vi "tm_startrecorder.vi"(8 "error in (no error)":errorcluster, 9 "frames":i32, 10 "File":path, 11 "Handle in":u32) -> (0 "error out":errorcluster, 3 "Handle out":u32)   [LabVIEW 2023]
uses:
  tmcamcon.dll
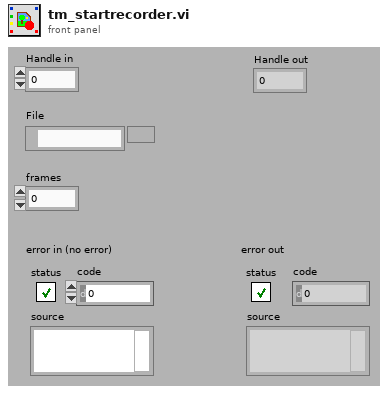
[diagram p1: front panel]
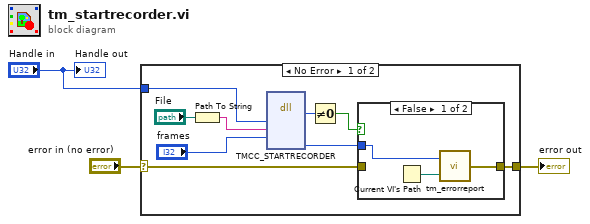
[diagram p0: block diagram]
diagram:
  n1 = case shown="No Error" "error in (no error)" {
    selector: "error in (no error)" -> [w7 w17]
    tunnel: [w4 w17] -> w2
    tunnel: "Handle in" -> [w11 _]
    frame No Error {
      n2 = Path To String(path="File") -> (string=w9:string)
      n3 = dll-call lib="tmcamcon.dll" fn="TMCC_STARTRECORDER"("handle"=w11, "path"=w9, "frames"="frames") -> ("return type"=w12:u32, "Erval"=w6:i32)  [unwired: 7 in, 2 out]
      n4 = Not Equal To 0?(x=w12) -> (x != 0?=w5:bool)
      n5 = case shown="False" w5 {
        tunnel: w7 -> [_ w16]
        tunnel: [w14 w16] -> w4
        tunnel: w6 -> [w13 _]
        frame False {
          n6 = Current VI's Path() -> (path=w15:path)
          n7 = call "tm_errorreport.vi"("Source"=w15, "Error"=w13) -> ("error out"=w14:errorcluster)
        }
        frame True {
        }
      }
    }
    frame Error {
    }
  }
  "error out" <- w2
  "Handle out" <- "Handle in"
